vi "GetADChannelsArray.vi"(8 "PXI6122Data":dbl[](array[numeric]), 9 "PXI6123Data":dbl[](array[numeric]), 10 "PXI6254Data":dbl[](array[numeric]), 11 "ADChannelStructArray":T1) -> (2 "ADChannelsArray":i16[](array[numeric]))   [LabVIEW 2011]
uses:
  ADChannelStructArray.ctl
  ADChannelStruct.ctl
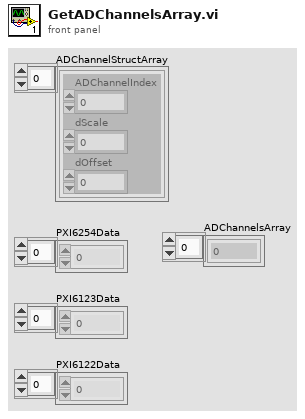
[diagram p1: front panel]
types:
  T1 = typedef "ADChannelStructArray.ctl" = T2[]
  T2 = typedef "ADChannelStruct.ctl" = cluster{"ADChannelIndex":i32, "dScale":dbl, "dOffset":dbl}
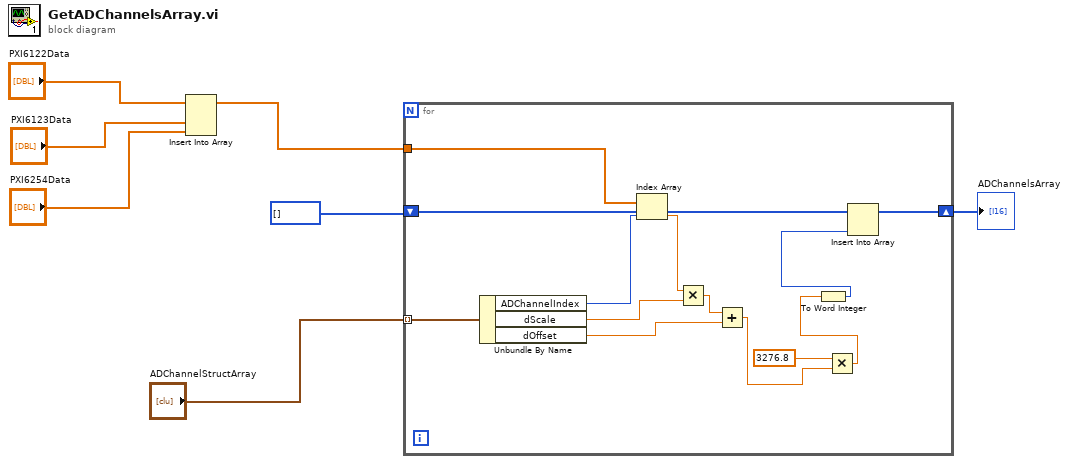
[diagram p0: block diagram]
diagram:
  n1 = Insert Into Array(array="PXI6122Data", new element #1="PXI6123Data", new element #2="PXI6254Data") -> (w1:dbl[])  [unwired: 1 in]
  n2 = for {
    tunnel: "ADChannelStructArray" -> [w20] mode=indexing
    tunnel: w1 -> [w19]
    shift-right: [w12] -> w5
    shift-left: u16[] [] -> [w17]
    n3 = Unbundle By Name(w20) -> ("ADChannelIndex"=w18:i32, "dScale"=w15:dbl, "dOffset"=w13:dbl)
    n4 = Index Array(array=w19, index=w18) -> (element=w16:dbl)
    n5 = Multiply(x=w16, y=w15) -> (x*y=w14:dbl)
    n6 = Add(x=w14, y=w13) -> (x+y=w8:dbl)
    n7 = Multiply(x=3276.8, y=w8) -> (x*y=w10:dbl)
    n8 = To Word Integer(number=w10) -> (16bit integer=w9:i16)
    n9 = Insert Into Array(array=w17, new element=w9) -> (w12:u16[])  [unwired: 1 in]
  }
  "ADChannelsArray" <- w5
